vi "F310.vi"(6 "error in (no error)":errorcluster, 7 "Deadzone Scale Cluster":cluster{"Scale":dbl, "Deadzone":dbl}, 8 "refnum name":string) -> (0 "Buttons":T2, 1 "D-Pad Buttons":T1, 2 "D-Pad":cluster{"X":dbl, "Y":dbl}, 3 "Right Stick":cluster{"X":dbl, "Y":dbl}, 4 "error out":errorcluster, 5 "Left Stick":cluster{"X":dbl, "Y":dbl})   [LabVIEW 2014]
uses:
  <vilib>/Rock Robotics/WPI/Joystick/WPI_JoystickGetSetRefNum.vi
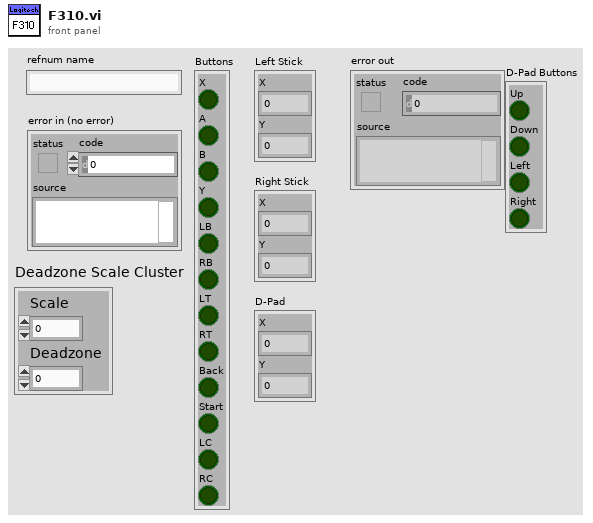
[diagram p1: front panel]
types:
  T1 = cluster{"Up":bool, "Down":bool, "Left":bool, "Right":bool}
  T2 = cluster{"X":bool, "A":bool, "B":bool, "Y":bool, "LB":bool, "RB":bool, "LT":bool, "RT":bool, "Back":bool, "Start":bool, "LC":bool, "RC":bool}
  T3 = typedef "WPI_JoystickDevRef.ctl" = cluster{"Device":T4}
  T4 = typedef "WPI_JoystickDeviceEnum.ctl" = enum16{"USB 0", "USB 1", "USB 2", "USB 3", "USB 4", "USB 5"}
  T5 = cluster{"Button 1":bool, "Button 2":bool, "Button 3":bool, "Button 4":bool, "Button 5":bool, "Button 6":bool, "Button 7":bool, "Button 8":bool, "Button 9":bool, "Button 10":bool, "Button 11":bool, "Button 12":bool}
  T6 = cluster{"axis 1 (x)":dbl, "axis 2 (y)":dbl, "axis 3 (throttle)":dbl, "axis 4":dbl, "axis 5":dbl, "axis 6":dbl}
  T7 = cluster{"[0]":dbl, "[1]":dbl, "[2]":dbl, "[3]":dbl, "[4]":dbl, "[5]":dbl}
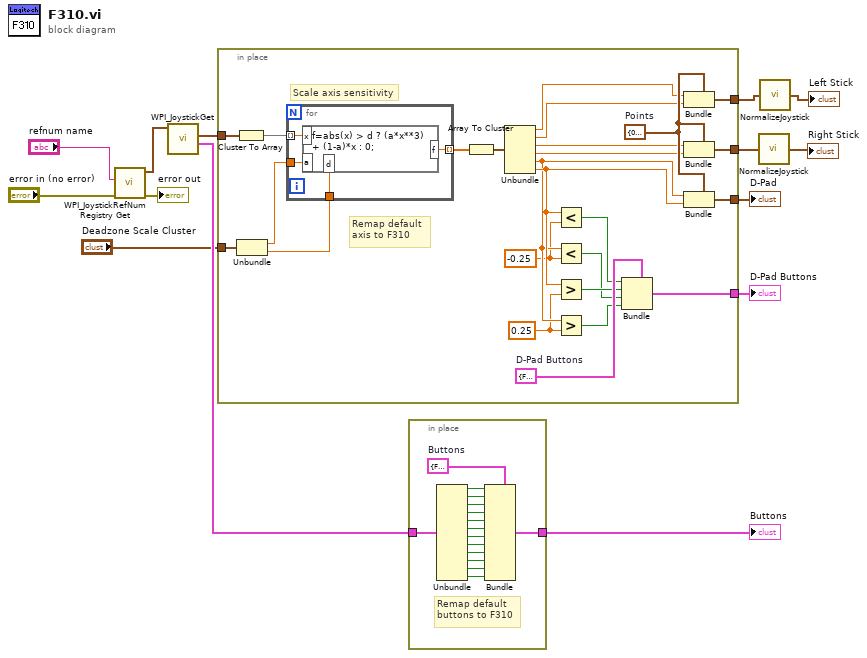
[diagram p0: block diagram]
diagram:
  n1 = call <vilib>:"WPI_JoystickRefNum Registry Get.vi"("error in (no error)"="error in (no error)", "refnum name"="refnum name") -> ("error out"=→"error out":errorcluster, "JoystickDevRef"=w14:T3)  [unwired: 8 in]
  n2 = call <vilib>:"WPI_JoystickGet.vi"("JoystickDevRef"=w14) -> ("Buttons"=w12:T5, "Axes"=w13:T6)  [unwired: 4 in, 1 out]
  n3 = in-place {
    in-place-border: w13 -> [w21]
    in-place-border: [w39] -> w4
    in-place-border: [w38] -> w2
    in-place-border: [w36] -> w8
    in-place-border: [w30] -> w6
    in-place-border: "Deadzone Scale Cluster" -> [w17]
    w31 = -0.25 ("y")
    w32 = 0.25 ("y")
    w35 = T1 {"Up"=FALSE, "Down"=FALSE, "Left"=FALSE, "Right"=FALSE}  # D-Pad Buttons
    w37 = cluster{"X":dbl, "Y":dbl} {"X"=0.0, "Y"=0.0}  # Points
    # "Scale axis sensitivity"
    # "Remap default\naxis to F310"
    n4 = Cluster To Array(cluster=w21) -> (array=w19:dbl[])
    n5 = Unbundle(w17) -> ("Scale"=w16:dbl, "Deadzone"=w15:dbl)
    n6 = for {
      tunnel: w19 -> [w43] mode=indexing
      tunnel: [w42] -> w18 mode=indexing
      tunnel: w16 -> [w41]
      tunnel: w15 -> [w40]
      n7 = formula code="f=abs(x) > d ? (a*x**3) + (1-a)*x : 0;"("x"=w43, "a"=w41, "d"=w40) -> ("f"=w42:dbl)
    }
    n8 = Array To Cluster(array=w18) -> (cluster=w20:T7)
    n9 = Unbundle(w20) -> ("[0]"=w25:dbl, "[1]"=w24:dbl, "[2]"=w23:dbl, "[3]"=w22:dbl, "[4]"=w33:dbl, "[5]"=w34:dbl)
    n10 = Less?(x=w34, y=w31) -> (x < y?=w28:bool)
    n11 = Less?(x=w33, y=w31) -> (x < y?=w26:bool)
    n12 = Greater?(x=w34, y=w32) -> (0:w29:bool)
    n13 = Greater?(x=w33, y=w32) -> (0:w27:bool)
    n14 = Bundle(cluster=w35, "Up"=w28, "Down"=w29, "Left"=w26, "Right"=w27) -> (w30:T1)
    n15 = Bundle(cluster=w37, "X"=w25, "Y"=w24) -> (w39:cluster{"X":dbl, "Y":dbl})
    n16 = Bundle(cluster=w37, "X"=w23, "Y"=w22) -> (w38:cluster{"X":dbl, "Y":dbl})
    n17 = Bundle(cluster=w37, "X"=w33, "Y"=w34) -> (w36:cluster{"X":dbl, "Y":dbl})
  }
  "D-Pad" <- w8
  "D-Pad Buttons" <- w6
  n18 = in-place {
    in-place-border: w12 -> [w58]
    in-place-border: [w44] -> w7
    w57 = T2 {"X"=FALSE, "A"=FALSE, "B"=FALSE, "Y"=FALSE, "LB"=FALSE, "RB"=FALSE, "LT"=FALSE, "RT"=FALSE, "Back"=FALSE, "Start"=FALSE, "LC"=FALSE, "RC"=FALSE}  # Buttons
    # "Remap default\nbuttons to F310"
    n19 = Unbundle(w58) -> ("Button 1"=w56:bool, "Button 2"=w55:bool, "Button 3"=w54:bool, "Button 4"=w53:bool, "Button 5"=w52:bool, "Button 6"=w51:bool, "Button 7"=w50:bool, "Button 8"=w49:bool, "Button 9"=w48:bool, "Button 10"=w47:bool, "Button 11"=w46:bool, "Button 12"=w45:bool)
    n20 = Bundle(cluster=w57, "X"=w56, "A"=w55, "B"=w54, "Y"=w53, "LB"=w52, "RB"=w51, "LT"=w50, "RT"=w49, "Back"=w48, "Start"=w47, "LC"=w46, "RC"=w45) -> (w44:T2)
  }
  "Buttons" <- w7
  n21 = call "NormalizeJoystick.vi"("joystick"=w2) -> ("normalized joystick"=→"Right Stick":cluster{"x":dbl, "y":dbl})
  n22 = call "NormalizeJoystick.vi"("joystick"=w4) -> ("normalized joystick"=→"Left Stick":cluster{"x":dbl, "y":dbl})
